vi "Generate Pulse Train.vi"(11 "O3 Frequency Train Actor in":refnum<class "O3 Frequency Train Actor.lvclass">) -> ()   [LabVIEW 2014]
uses:
  <vilib>/Platform/TimedLoop/XDataNode/wakeup.ctl
  <vilib>/Platform/TimedLoop/XDataNode/XDNodeRunTimeDep.lvlib
  <vilib>/Platform/TimedLoop/XDataNode/nitl_modes.ctl
  <vilib>/Platform/TimedLoop/XDataNode/timing_clust.ctl
  <vilib>/Platform/TimedLoop/XDataNode/XDataNode.xnode
  <vilib>/DAQmx/write.llb/DAQmx Write (Digital Bool 1Line 1Point).vi
  O3 Frequency Train Actor.lvclass
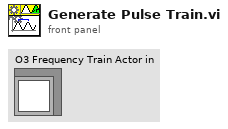
[diagram p1: front panel]
types:
  T1 = typedef "XDNodeRunTimeDep.lvlib/nitl_modes.ctl" = enum32{"No Change", "Process missed periods, maintain original phase", "Discard missed periods, maintain original phase", "Process missed periods, ignore original phase", "Discard missed periods, ignore original phase"}
  T2 = typedef "XDNodeRunTimeDep.lvlib/timing_clust.ctl" = cluster{"Expected End [f-1]":u64, "Actual End [f-1]":u64, "Finished Late? [f-1]":bool, "Expected End [i-1]":u64, "Actual End [i-1]":u64, "Finished Late? [i-1]":bool, "Expected Start [i]":u64, "Actual Start [i]":u64, "Expected Start [f]":u64, "Actual Start [f]":u64, "Source Name":string, "Structure Name":string, "Period":i64, "Deadline":i64, "Offset":i64, "Start":i64, "Priority":i32, "Timeout":i32, "Mode":T1, "Wakeup Reason":T3, "Error":errorcluster, "Source Type":string, "Secondary Source Type":string, "Global End Time":u64, "Global Start Time":u64, "Frame Duration":u64, "Iteration Duration":u64, "Assigned CPU":i32, "I/O Scan Engine Mode":u32}
  T3 = typedef "XDNodeRunTimeDep.lvlib/wakeup.ctl" = enum32{"Normal", "Aborted", "Asynchronous wakeup", "Timing source error", "Timed loop error", "Timeout"}
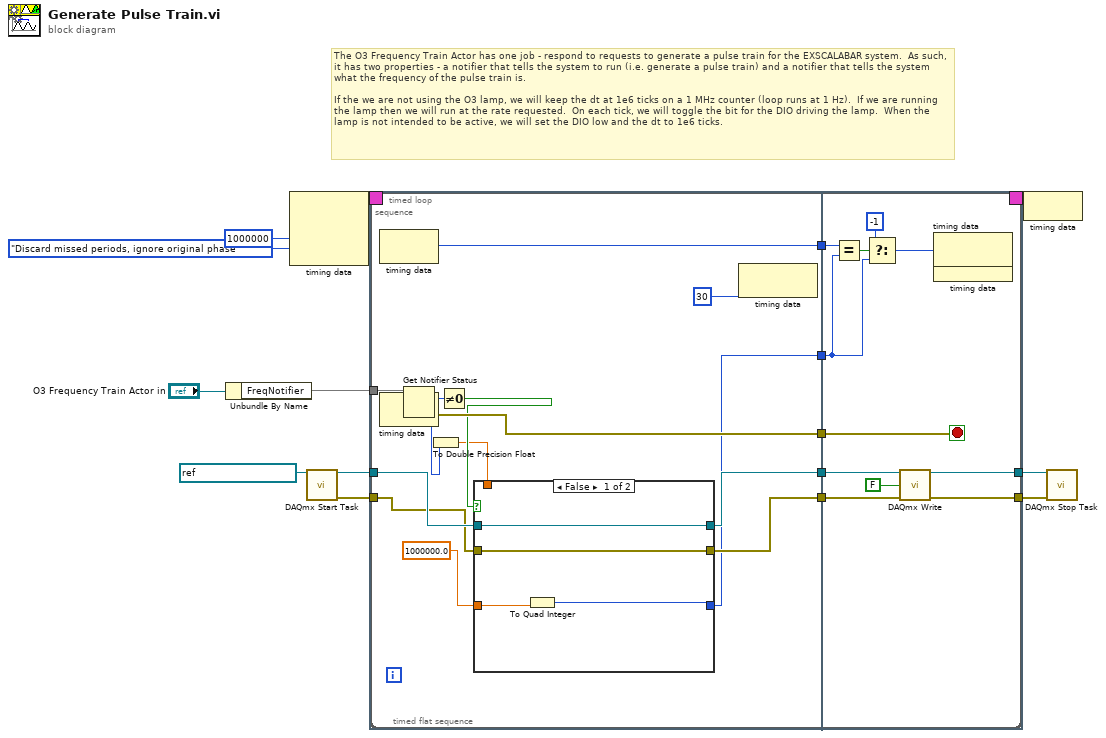
[diagram p0: block diagram]
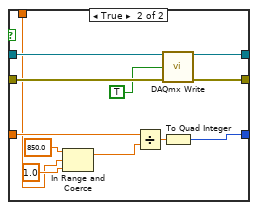
[diagram p2: hidden frame]
diagram:
  # "The O3 Frequency Train Actor has one job - respond to requests to generate a pulse train for the EXSCALABAR system.  As such, it has two properties - a notifier that tells the system to run (i.e. generate a pulse train) and a notifier that tells the system what the frequency of the pulse train is.  \n\nIf the we are not using the O3 lamp, we will keep the dt at 1e6 ticks on a 1 MHz counter (loop runs at 1 Hz).  If we are running the lamp then we will run at the rate requested.  On each tick, we will toggle the bit for the DIO driving the lamp.  When the lamp is not intended to be active, we will set the DIO low and the dt to 1e6 ticks."
  n1 = Unbundle By Name("O3 Frequency Train Actor in") -> ("FreqNotifier"=w4)
  n2 = node-c288(i64 1000000 ("Period"), nitl_modes."Discard missed periods, ignore original phase" ("Mode")) -> (w11:T2)  [unwired: 1 in]
  n3 = call <vilib>:"DAQmx Start Task.vi"("task/channels in"=refnum<k21> "O3 Lamp Output") -> ("task out"=w8:refnum<k21>, "error out"=w6:errorcluster)  [unwired: 13 in]
  n4 = timed-loop {
    timing: w11 -> [_]
    timing-out: [_] -> w10
    tunnel: w8 -> [w16]
    tunnel: [w15] -> w9
    tunnel: w6 -> [w14]
    tunnel: [w13] -> w5
    tunnel: w4 -> [w12]
    stop <- w62 stop-if-true
    n5 = timed-sequence {
      timing: _ -> [_]
      timing-out: _ -> [_]
      tunnel: w16 -> [w26]
      tunnel: [w25] -> w15
      tunnel: w14 -> [w24]
      tunnel: [w23] -> w13
      tunnel: w12 -> [w17]
      n6 = timed-flat-sequence {
        tunnel: w26 -> [w39]
        tunnel: w24 -> [w38]
        tunnel: [w36] -> w22
        tunnel: [w37] -> w21
        tunnel: [w33] -> w20
        tunnel: [w31] -> w19
        tunnel: [w35] -> w18
        tunnel: w17 -> [w34]
        tunnel: [w68] -> w23
        tunnel: [w70] -> w25
        tunnel: w22 -> [w71]
        tunnel: w21 -> [w69]
        tunnel: w20 -> [w65]
        tunnel: w19 -> [w63]
        tunnel: w18 -> [w62]
        frame #0 {
          n7 = node-c288() -> (w33:i64)  [unwired: 1 in]
          n8 = Get Notifier Status(notifier=w34) -> (current notification=w28:i64, error out=w35:errorcluster)  [unwired: 1 in, 3 out]
          n9 = To Double Precision Float(number=w28) -> (double precision float=w27:dbl)
          n10 = Not Equal To 0?(x=w28) -> (x != 0?=w30:bool)
          n11 = case shown="False" w30 {
            tunnel: w39 -> [w43 w55]
            tunnel: w38 -> [w42 w54]
            tunnel: [w42 w53] -> w37
            tunnel: [w43 w52] -> w36
            tunnel: [w40 w49] -> w31
            tunnel: 1000000.0 ("x") -> [w41 w48]
            tunnel: w27 -> [_ w44]
            frame False {
              n12 = To Quad Integer(1:w41) -> (0:w40:i64)
            }
            frame True {
              n13 = In Range and Coerce(upper limit=850.0, x=w44, lower limit=1.0) -> (coerced(x)=w46:dbl)  [unwired: 1 out]
              n14 = Divide(x=w48, y=w46) -> (x/y=w50:dbl)
              n15 = call-poly <vilib>:"DAQmx Write.vi"("task/channels in"=w55, "data"=TRUE ("auto start"), "error in"=w54) -> ("task out"=w52:refnum<k21>, "error out"=w53:errorcluster)  [unwired: 10 in, 1 out]
              n16 = To Quad Integer(1:w50) -> (0:w49:i64)
            }
          }
          n17 = node-c288(i64 30 ("Pulse width")) -> ()  [unwired: 1 out]
        }
        frame #1 {
          n18 = Equal?(x=w65, y=w63) -> (x = y?=w66:bool)
          n19 = Select(t=i64 -1, s=w66, f=w63) -> (s? t:f=w64:i64)
          n20 = call-poly <vilib>:"DAQmx Write.vi"("task/channels in"=w71, "data"=FALSE, "error in"=w69) -> ("task out"=w70:refnum<k21>, "error out"=w68:errorcluster)  [unwired: 10 in, 1 out]
          n21 = node-c288(w64) -> ()  [unwired: 1 out]
        }
      }
    }
    n22 = node-c288() -> ()  [unwired: 1 in, 1 out]
    n23 = node-c288() -> ()  [unwired: 1 in, 1 out]
  }
  n24 = node-c288(w10) -> ()
  n25 = call <vilib>:"DAQmx Stop Task.vi"("task/channels in"=w9, "error in"=w5) -> ()  [unwired: 12 in, 2 out]
